vi "Custom Aggregation (Power Values).vi"(0 "power values":T3, 1 "reset? (F)":bool, 5 "aggregation settings":T1={"interval"=1, "interval unit"=enum."Runs", "synchronization of intervals"=enum."Not synchronized", "algorithm"=enum."Average"}, 9 "system info in":refnum<class "EP System Info.lvclass">, 11 "error in (no error)":errorcluster, 12 "data timestamp":timestamp) -> (4 "aggregated minimum value":T3, 6 "aggregated averaged/RMS value":T3, 8 "aggregated maximum value":T2, 10 "system info out":refnum<class "EP System Info.lvclass">, 13 "aggregated data valid?":bool, 14 "aggregated data timestamp":timestamp, 15 "error out":errorcluster)   [LabVIEW 2014, in "NI_EP_Power Quality.lvlib"]
doc: "Calculates the aggregated minimum, maximum, and averaged or RMS value of an input signal for a specified aggregation interval, according to Class S in IEC 61000-4-30:2008. There is no overlap between aggregation intervals. This VI automatically restarts accumulation at the beginning of the next time interval after the previous interval expires. You must manually select the polymorphic instance you want to use.\n\nThis VI supports measuring single-line and multiple-line systems except the DBL instance. Use the DBL instance to measure one channel on one line at one time."
uses:
  <vilib>/addons/Electrical Power/PQ/NI_EP_Power Quality.lvlib
  <vilib>/addons/Electrical Power/PQ/Common/Controls/ep_Aggregation Settings.ctl
  <vilib>/addons/Electrical Power/PQ/Common/Classes/System Info/EP System Info.lvclass
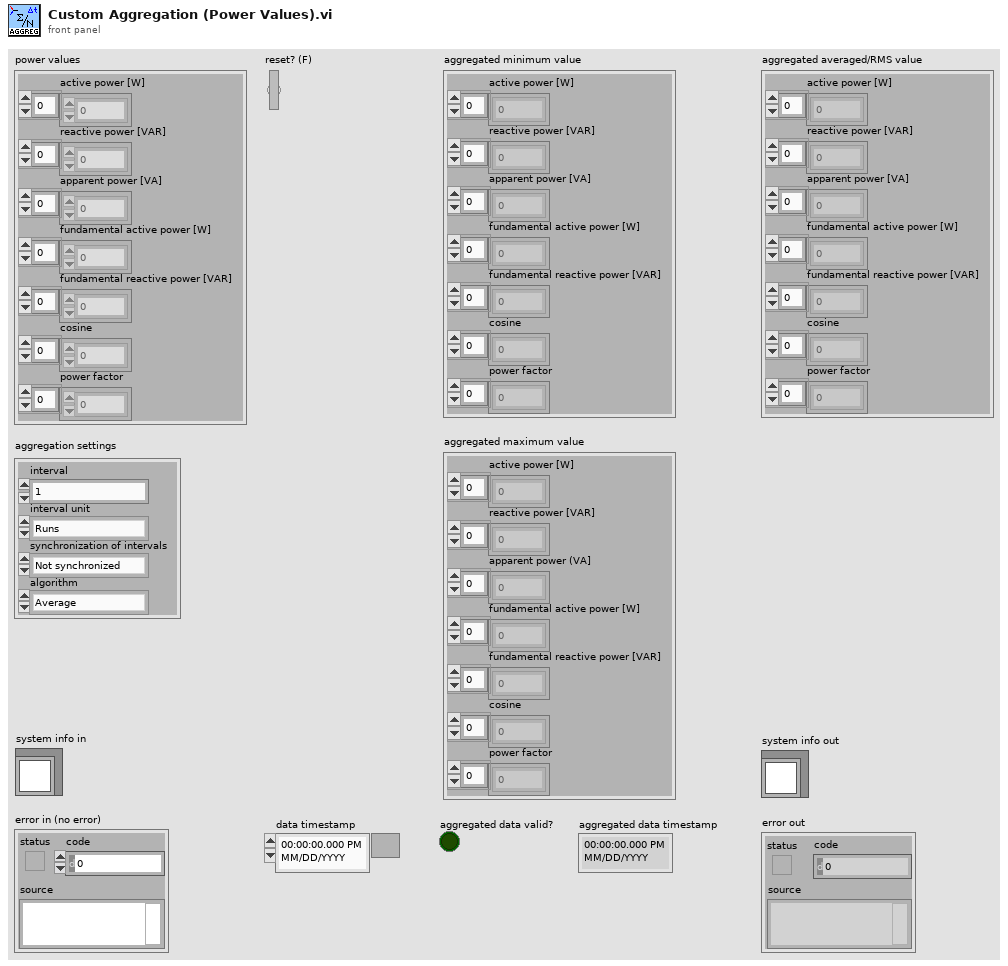
[diagram p1: front panel]
types:
  T1 = typedef "NI_EP_Power Quality.lvlib/ep_Aggregation Settings.ctl" = cluster{"interval":u32, "interval unit":enum16{"Runs", "Seconds", "Minutes", "Hours", "Days", "Weeks"}, "synchronization of intervals":enum16{"Not synchronized", "Interval rounded"}, "algorithm":enum16{"Average", "RMS"}}
  T2 = cluster{"active power [W]":dbl[], "reactive power [VAR]":dbl[], "apparent power (VA]":dbl[], "fundamental active power [W]":dbl[], "fundamental reactive power [VAR]":dbl[], "cosine":dbl[], "power factor":dbl[]}
  T3 = cluster{"active power [W]":dbl[], "reactive power [VAR]":dbl[], "apparent power [VA]":dbl[], "fundamental active power [W]":dbl[], "fundamental reactive power [VAR]":dbl[], "cosine":dbl[], "power factor":dbl[]}
  T4 = cluster{"aggregated minimum values":dbl[], "aggregated minimum values":dbl[], "aggregated minimum values":dbl[], "aggregated minimum values":dbl[], "aggregated minimum values":dbl[], "aggregated minimum values":dbl[], "aggregated minimum values":dbl[]}
  T5 = cluster{"aggregated averaged/RMS values":dbl[], "aggregated averaged/RMS values":dbl[], "aggregated averaged/RMS values":dbl[], "aggregated averaged/RMS values":dbl[], "aggregated averaged/RMS values":dbl[], "aggregated averaged/RMS values":dbl[], "aggregated averaged/RMS values":dbl[]}
  T6 = cluster{"aggregated maximum values":dbl[], "aggregated maximum values":dbl[], "aggregated maximum values":dbl[], "aggregated maximum values":dbl[], "aggregated maximum values":dbl[], "aggregated maximum values":dbl[], "aggregated maximum values":dbl[]}
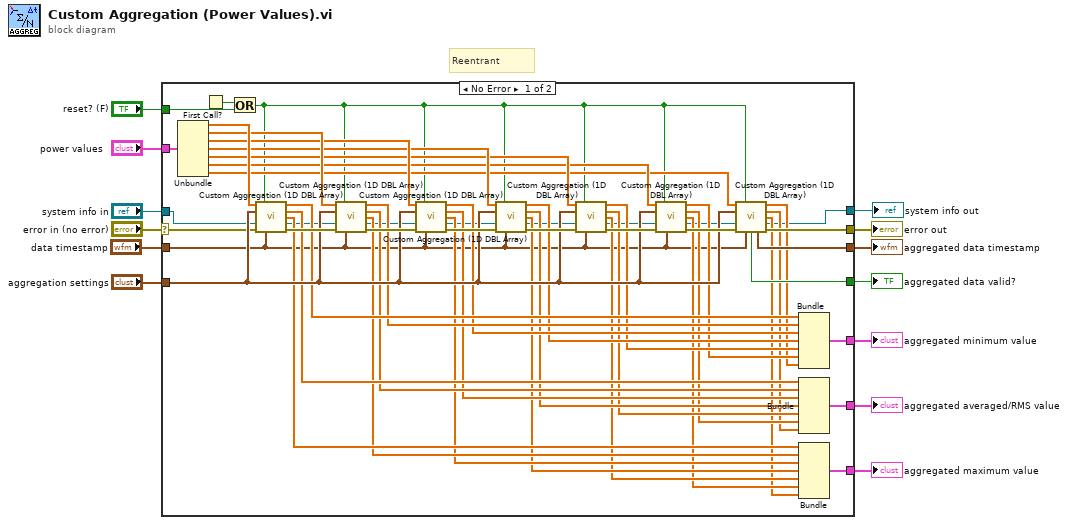
[diagram p0: block diagram]
diagram:
  # "Reentrant"
  n1 = case shown="No Error" "error in (no error)" {
    selector: "error in (no error)" -> [w26 w70]
    tunnel: "power values" -> [w68 _]
    tunnel: "reset? (F)" -> [w24 _]
    tunnel: [w61 w70] -> w11
    tunnel: [w60 _] -> w10
    tunnel: [w59 _] -> w9
    tunnel: [w58 _] -> w8
    tunnel: [w57 _] -> w4
    tunnel: "aggregation settings" -> [w49 _]
    tunnel: [w48 _] -> w3
    tunnel: "data timestamp" -> [w22 _]
    tunnel: "system info in" -> [w21 w69]
    tunnel: [w14 w69] -> w1
    frame No Error {
      n2 = Unbundle(w68) -> ("active power [W]"=w56:dbl[], "reactive power [VAR]"=w55:dbl[], "apparent power [VA]"=w54:dbl[], "fundamental active power [W]"=w53:dbl[], "fundamental reactive power [VAR]"=w52:dbl[], "cosine"=w51:dbl[], "power factor"=w50:dbl[])
      n3 = First Call?() -> (First Call?: T/F=w25:bool)
      n4 = Or(x=w25, y=w24) -> (x .or. y?=w23:bool)
      n5 = call <vilib>:"Custom Aggregation (1D DBL Array).vi"("data in"=w56, "reset? (F)"=w23, "aggregation settings"=w49, "system info in"=w21, "error in (no error)"=w26, "data timestamp"=w22) -> ("aggregated minimum values"=w47:dbl[], "aggregated averaged/RMS values"=w40:dbl[], "aggregated maximum values"=w33:dbl[], "system info out"=w20:refnum<class "EP System Info.lvclass">, "error out"=w67:errorcluster)  [unwired: 3 in, 2 out]
      n6 = call <vilib>:"Custom Aggregation (1D DBL Array).vi"("data in"=w55, "reset? (F)"=w23, "aggregation settings"=w49, "system info in"=w20, "error in (no error)"=w67, "data timestamp"=w22) -> ("aggregated minimum values"=w46:dbl[], "aggregated averaged/RMS values"=w39:dbl[], "aggregated maximum values"=w32:dbl[], "system info out"=w19:refnum<class "EP System Info.lvclass">, "error out"=w66:errorcluster)  [unwired: 3 in, 2 out]
      n7 = call <vilib>:"Custom Aggregation (1D DBL Array).vi"("data in"=w54, "reset? (F)"=w23, "aggregation settings"=w49, "system info in"=w19, "error in (no error)"=w66, "data timestamp"=w22) -> ("aggregated minimum values"=w45:dbl[], "aggregated averaged/RMS values"=w38:dbl[], "aggregated maximum values"=w31:dbl[], "system info out"=w18:refnum<class "EP System Info.lvclass">, "error out"=w65:errorcluster)  [unwired: 3 in, 2 out]
      n8 = call <vilib>:"Custom Aggregation (1D DBL Array).vi"("data in"=w53, "reset? (F)"=w23, "aggregation settings"=w49, "system info in"=w18, "error in (no error)"=w65, "data timestamp"=w22) -> ("aggregated minimum values"=w44:dbl[], "aggregated averaged/RMS values"=w37:dbl[], "aggregated maximum values"=w30:dbl[], "system info out"=w17:refnum<class "EP System Info.lvclass">, "error out"=w64:errorcluster)  [unwired: 3 in, 2 out]
      n9 = call <vilib>:"Custom Aggregation (1D DBL Array).vi"("data in"=w52, "reset? (F)"=w23, "aggregation settings"=w49, "system info in"=w17, "error in (no error)"=w64, "data timestamp"=w22) -> ("aggregated minimum values"=w43:dbl[], "aggregated averaged/RMS values"=w36:dbl[], "aggregated maximum values"=w29:dbl[], "system info out"=w16:refnum<class "EP System Info.lvclass">, "error out"=w63:errorcluster)  [unwired: 3 in, 2 out]
      n10 = call <vilib>:"Custom Aggregation (1D DBL Array).vi"("data in"=w51, "reset? (F)"=w23, "aggregation settings"=w49, "system info in"=w16, "error in (no error)"=w63, "data timestamp"=w22) -> ("aggregated minimum values"=w42:dbl[], "aggregated averaged/RMS values"=w35:dbl[], "aggregated maximum values"=w28:dbl[], "system info out"=w15:refnum<class "EP System Info.lvclass">, "error out"=w62:errorcluster)  [unwired: 3 in, 2 out]
      n11 = call <vilib>:"Custom Aggregation (1D DBL Array).vi"("data in"=w50, "reset? (F)"=w23, "aggregation settings"=w49, "system info in"=w15, "error in (no error)"=w62, "data timestamp"=w22) -> ("aggregated minimum values"=w41:dbl[], "aggregated averaged/RMS values"=w34:dbl[], "aggregated maximum values"=w27:dbl[], "system info out"=w14:refnum<class "EP System Info.lvclass">, "aggregated data valid?"=w48:bool, "aggregated data timestamp"=w57:timestamp, "error out"=w61:errorcluster)  [unwired: 3 in]
      n12 = Bundle("aggregated minimum values"=w47, "aggregated minimum values"=w46, "aggregated minimum values"=w45, "aggregated minimum values"=w44, "aggregated minimum values"=w43, "aggregated minimum values"=w42, "aggregated minimum values"=w41) -> (w60:T4)  [unwired: 1 in]
      n13 = Bundle("aggregated averaged/RMS values"=w40, "aggregated averaged/RMS values"=w39, "aggregated averaged/RMS values"=w38, "aggregated averaged/RMS values"=w37, "aggregated averaged/RMS values"=w36, "aggregated averaged/RMS values"=w35, "aggregated averaged/RMS values"=w34) -> (w59:T5)  [unwired: 1 in]
      n14 = Bundle("aggregated maximum values"=w33, "aggregated maximum values"=w32, "aggregated maximum values"=w31, "aggregated maximum values"=w30, "aggregated maximum values"=w29, "aggregated maximum values"=w28, "aggregated maximum values"=w27) -> (w58:T6)  [unwired: 1 in]
    }
    frame Error {
    }
  }
  "error out" <- w11
  "aggregated minimum value" <- w10
  "aggregated averaged/RMS value" <- w9
  "aggregated maximum value" <- w8
  "aggregated data valid?" <- w3
  "aggregated data timestamp" <- w4
  "system info out" <- w1
